vi "PluginCore GetStatusData.vi"(6 "contextId":T1, 8 "error in":errorcluster, 9 "timeout (ms)":i32=-1, 10 "Request Data":T11, 11 "gRPC ID":T1) -> (0 "error out":errorcluster, 2 "Response Data":T2, 3 "gRPC ID out":T1)   [LabVIEW 2021, in "CIFCorePlugin_client.lvlib"]
uses:
  CIFCorePlugin_client.lvlib
  <vilib>/gRPC/LabVIEW gRPC Library/Shared/grpcId.ctl
  RPC Messages/cif_common_Empty.ctl
  RPC Messages/cif_plugincore_StatusData.ctl
  RPC Messages/cif_plugincore_StatusData_State.ctl
  RPC Messages/cif_plugincore_TimingStatistics.ctl
  RPC Messages/cif_common_TimingStats.ctl
  RPC Messages/cif_plugincore_FifoStatistics.ctl
  RPC Messages/cif_plugincore_Error.ctl
  RPC Messages/cif_plugincore_MonitorDoubles.ctl
  RPC Messages/cif_plugincore_MonitorU64.ctl
  RPC Messages/cif_plugincore_MonitorI64.ctl
  RPC Messages/cif_plugincore_StatusData_Flat.ctl
  RPC Messages/cif_plugincore_TimingStatistics_Flat.ctl
  RPC Messages/cif_common_TimingStats_Flat.ctl
  RPC Messages/cif_plugincore_FifoStatistics_Flat.ctl
  RPC Messages/cif_plugincore_Error_Flat.ctl
  RPC Messages/cif_plugincore_MonitorDoubles_Flat.ctl
  RPC Messages/cif_plugincore_MonitorU64_Flat.ctl
  RPC Messages/cif_plugincore_MonitorI64_Flat.ctl
  14035477-4c25-4107-8ed5-d0c4ef420ce5.vi
  <vilib>/gRPC/LabVIEW gRPC Library/Shared/TranslateGrpcError.vi
  <vilib>/gRPC/LabVIEW gRPC Library/Shared/Wait On Occurrence Wrapper.vi
  RPC Messages/FlatToRichcif_plugincore_TimingStatistics.vi
  RPC Messages/FlatToRichcif_plugincore_FifoStatistics.vi
  RPC Messages/FlatToRichcif_plugincore_Error.vi
  RPC Messages/FlatToRichcif_plugincore_MonitorDoubles.vi
  RPC Messages/FlatToRichcif_plugincore_MonitorU64.vi
  RPC Messages/FlatToRichcif_plugincore_MonitorI64.vi
  <vilib>/gRPC/LabVIEW gRPC Library/Shared/Wait On Occurence.vi
  RPC Messages/FlatToRichcif_common_TimingStats.vi
  <vilib>/gRPC/LabVIEW gRPC Library/Server API/Server/Get Server DLL Path.vi
  <vilib>/Utility/error.llb/Error Cluster From Error Code.vi
  <vilib>/Utility/config.llb/Open Config Data.vi
  <vilib>/Utility/config.llb/Write Key.vi
  <vilib>/Utility/config.llb/Write Key (Boolean).vi
  <vilib>/Utility/config.llb/Not A Config Data Refnum.vi
  <vilib>/Utility/config.llb/Read Key.vi
  <vilib>/Utility/config.llb/Read Key (Boolean).vi
  <vilib>/Utility/config.llb/Close Config Data.vi
  <vilib>/gRPC/LabVIEW gRPC Library/grpc-lvsupport-release.lvlib
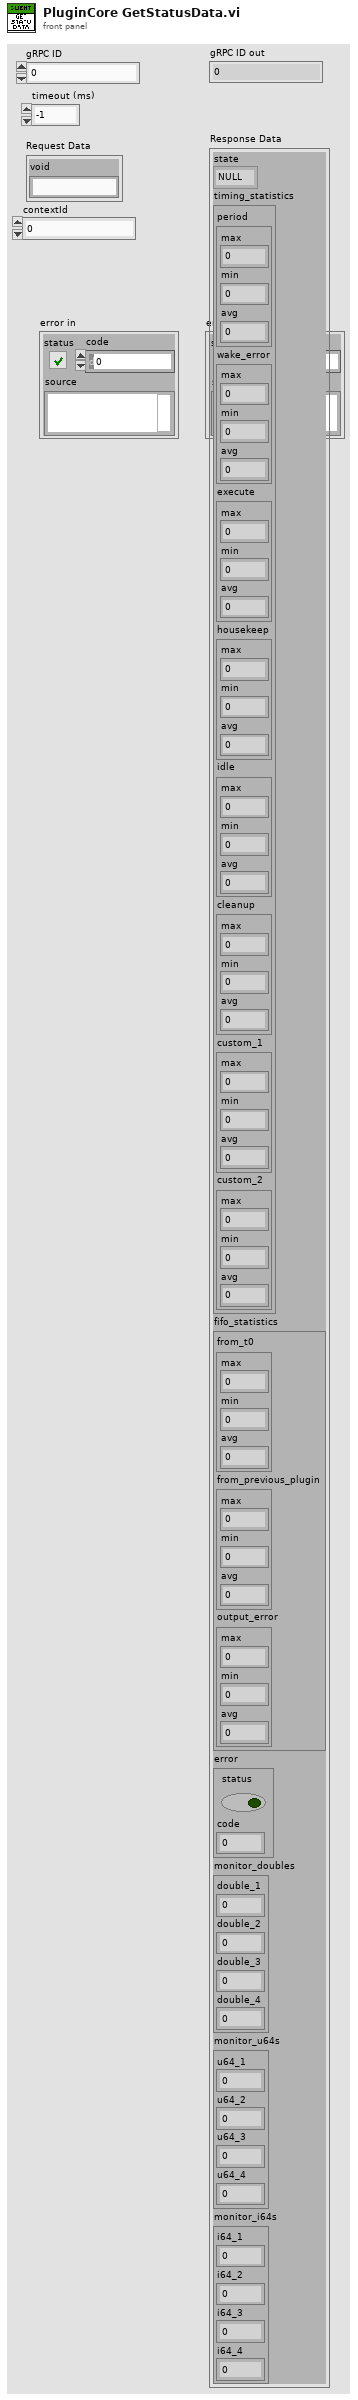
[diagram p1: front panel]
types:
  T1 = typedef "grpc-lvsupport-release.lvlib/grpcId.ctl" = u64
  T2 = typedef "CIFCorePlugin_client.lvlib/cif_plugincore_StatusData.ctl" = cluster{"state":T3, "timing_statistics":T4, "fifo_statistics":T6, "error":T7, "monitor_doubles":T8, "monitor_u64s":T9, "monitor_i64s":T10}
  T3 = typedef "CIFCorePlugin_client.lvlib/cif_plugincore_StatusData_State.ctl" = enum32{"NULL", "CREATING", "LISTENING", "RUNNING", "CLEANINGUP", "DESTROYING"}
  T4 = typedef "CIFCorePlugin_client.lvlib/cif_plugincore_TimingStatistics.ctl" = cluster{"period":T5, "wake_error":T5, "execute":T5, "housekeep":T5, "idle":T5, "cleanup":T5, "custom_1":T5, "custom_2":T5}
  T5 = typedef "CIFCorePlugin_client.lvlib/cif_common_TimingStats.ctl" = cluster{"max":i64, "min":i64, "avg":dbl}
  T6 = typedef "CIFCorePlugin_client.lvlib/cif_plugincore_FifoStatistics.ctl" = cluster{"from_t0":T5, "from_previous_plugin":T5, "output_error":T5}
  T7 = typedef "CIFCorePlugin_client.lvlib/cif_plugincore_Error.ctl" = cluster{"status":bool, "code":i32}
  T8 = typedef "CIFCorePlugin_client.lvlib/cif_plugincore_MonitorDoubles.ctl" = cluster{"double_1":dbl, "double_2":dbl, "double_3":dbl, "double_4":dbl}
  T9 = typedef "CIFCorePlugin_client.lvlib/cif_plugincore_MonitorU64.ctl" = cluster{"u64_1":u64, "u64_2":u64, "u64_3":u64, "u64_4":u64}
  T10 = typedef "CIFCorePlugin_client.lvlib/cif_plugincore_MonitorI64.ctl" = cluster{"i64_1":i64, "i64_2":i64, "i64_3":i64, "i64_4":i64}
  T11 = typedef "CIFCorePlugin_client.lvlib/cif_common_Empty.ctl" = cluster{"void":string}
  T12 = typedef "CIFCorePlugin_client.lvlib/cif_plugincore_StatusData_Flat.ctl" = cluster{"state":T3, "timing_statistics":T13, "fifo_statistics":T15, "error":T16, "monitor_doubles":T17, "monitor_u64s":T18, "monitor_i64s":T19}
  T13 = typedef "CIFCorePlugin_client.lvlib/cif_plugincore_TimingStatistics_Flat.ctl" = cluster{"period":T14, "wake_error":T14, "execute":T14, "housekeep":T14, "idle":T14, "cleanup":T14, "custom_1":T14, "custom_2":T14}
  T14 = typedef "CIFCorePlugin_client.lvlib/cif_common_TimingStats_Flat.ctl" = cluster{"max":i64, "min":i64, "avg":dbl}
  T15 = typedef "CIFCorePlugin_client.lvlib/cif_plugincore_FifoStatistics_Flat.ctl" = cluster{"from_t0":T14, "from_previous_plugin":T14, "output_error":T14}
  T16 = typedef "CIFCorePlugin_client.lvlib/cif_plugincore_Error_Flat.ctl" = cluster{"status":bool, "code":i32}
  T17 = typedef "CIFCorePlugin_client.lvlib/cif_plugincore_MonitorDoubles_Flat.ctl" = cluster{"double_1":dbl, "double_2":dbl, "double_3":dbl, "double_4":dbl}
  T18 = typedef "CIFCorePlugin_client.lvlib/cif_plugincore_MonitorU64_Flat.ctl" = cluster{"u64_1":u64, "u64_2":u64, "u64_3":u64, "u64_4":u64}
  T19 = typedef "CIFCorePlugin_client.lvlib/cif_plugincore_MonitorI64_Flat.ctl" = cluster{"i64_1":i64, "i64_2":i64, "i64_3":i64, "i64_4":i64}
  T20 = typedef "CIFCorePlugin_client.lvlib/cif_common_Empty_Flat.ctl" = cluster{"void":string}
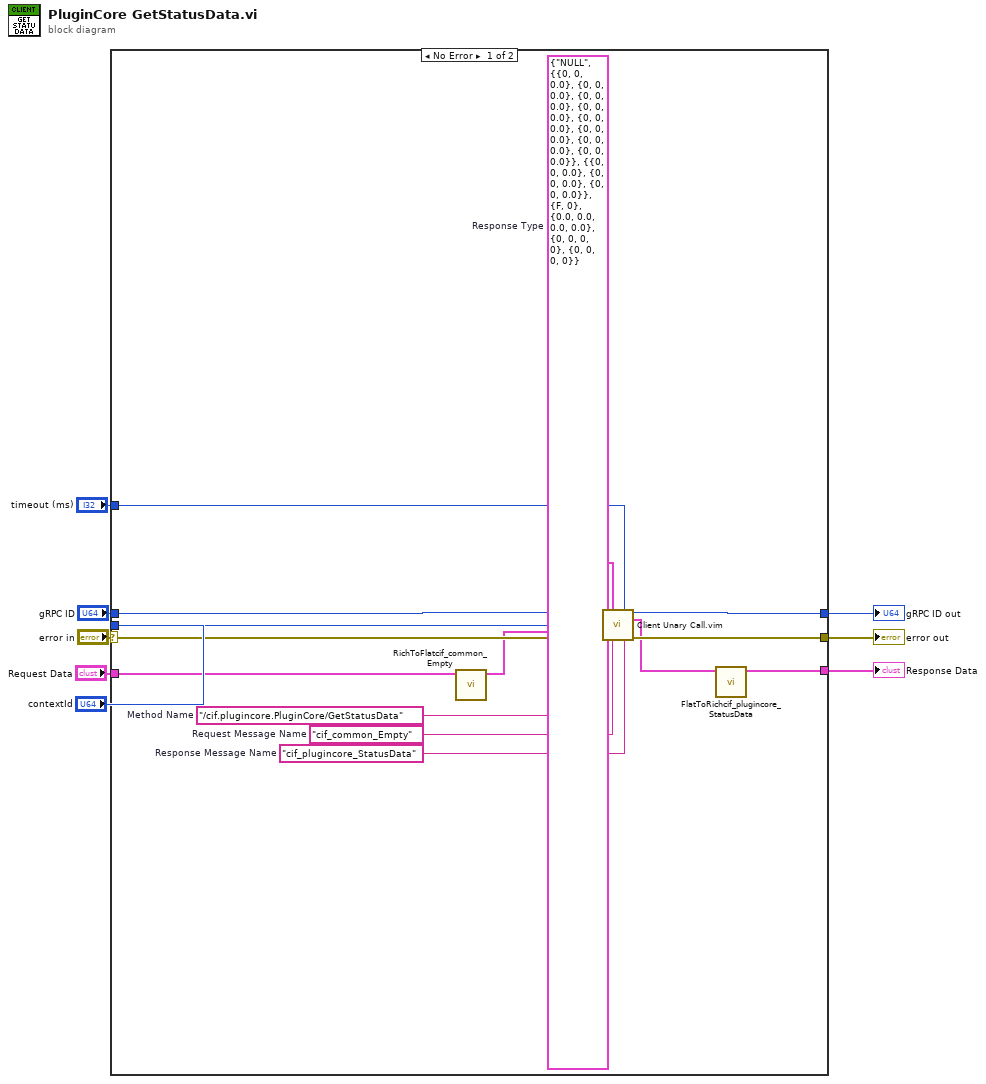
[diagram p0: block diagram]
diagram:
  n1 = case shown="No Error" "error in" {
    selector: "error in" -> [w18 w23]
    tunnel: [w17 w23] -> w7
    tunnel: "gRPC ID" -> [w16 w24]
    tunnel: [w15 w24] -> w5
    tunnel: "Request Data" -> [w12 _]
    tunnel: [w9 _] -> w3
    tunnel: "timeout (ms)" -> [w14 _]
    tunnel: "contextId" -> [w13 _]
    frame No Error {
      w19 = "cif_plugincore_StatusData"  # Response Message Name
      w20 = "cif_common_Empty"  # Request Message Name
      w21 = T12 {"state"=enum."NULL", "timing_statistics"={"period"={"max"=0, "min"=0, "avg"=0.0}, "wake_error"={"max"=0, "min"=0, "avg"=0.0}, "execute"={"max"=0, "min"=0, "avg"=0.0}, "housekeep"={"max"=0, "min"=0, "avg"=0.0}, "idle"={"max"=0, "min"=0, "avg"=0.0}, "cleanup"={"max"=0, "min"=0, "avg"=0.0}, "custom_1"={"max"=0, "min"=0, "avg"=0.0}, "custom_2"={"max"=0, "min"=0, "avg"=0.0}}, "fifo_statistics"={"from_t0"={"max"=0, "min"=0, "avg"=0.0}, "from_previous_plugin"={"max"=0, "min"=0, "avg"=0.0}, "output_error"={"max"=0, "min"=0, "avg"=0.0}}, "error"={"status"=FALSE, "code"=0}, "monitor_doubles"={"double_1"=0.0, "double_2"=0.0, "double_3"=0.0, "double_4"=0.0}, "monitor_u64s"={"u64_1"=0, "u64_2"=0, "u64_3"=0, "u64_4"=0}, "monitor_i64s"={"i64_1"=0, "i64_2"=0, "i64_3"=0, "i64_4"=0}}  # Response Type
      w22 = "/cif.plugincore.PluginCore/GetStatusData"  # Method Name
      n2 = call "RichToFlatcif_common_Empty.vi"("InputCluster"=w12) -> ("OutputCluster"=w11:T20)  [unwired: 10 in]
      n3 = call "Client Unary Call.vim"("ClientID in"=w16, "Response Type"=w21, "timeout (ms)"=w14, "Method Name"=w22, "contextId"=w13, "Request Data"=w11, "error in"=w18, "Request Message Name"=w20, "Response Message Name"=w19) -> ("ClientID out"=w15:u64, "Response Data"=w10:T12, "error out"=w17:errorcluster)  [unwired: 4 in]
      n4 = call "FlatToRichcif_plugincore_StatusData.vi"("InputCluster"=w10) -> ("OutputCluster"=w9:T2)  [unwired: 10 in]
    }
    frame Error {
    }
  }
  "error out" <- w7
  "gRPC ID out" <- w5
  "Response Data" <- w3
